vi "string_to_array.vi"(10 "String":string) -> (2 "Array":string[](array[string]))   [LabVIEW 2018]
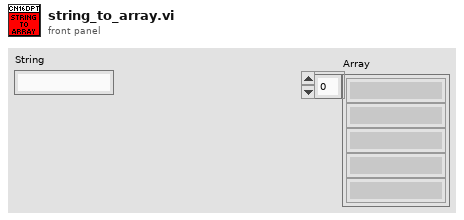
[diagram p1: front panel]
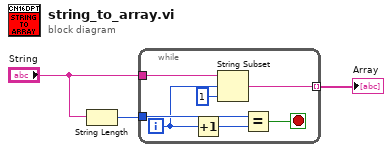
[diagram p0: block diagram]
diagram:
  n1 = String Length(string="String") -> (length=w1:i32)
  n2 = while {
    tunnel: "String" -> [w10]
    tunnel: [w9] -> w3 mode=indexing
    tunnel: w1 -> [w8]
    i -> [w4]
    stop <- w7 stop-if-true
    n3 = Increment(x=w4) -> (x+1=w5:i32)
    n4 = String Subset(string=w10, offset (0)=w4, length (rest)=1 ("length (rest)")) -> (substring=w9:string)
    n5 = Equal?(x=w8, y=w5) -> (x = y?=w7:bool)
  }
  "Array" <- w3
